vi "ReadINIandWriteToGFG.vi"(8 "error in (no error)":errorcluster, 10 "name or relative path":string="settings.ini", 11 "configuration file path":path) -> (0 "error out":errorcluster)   [LabVIEW 2012]
doc: "This VI reads an INI file and stores all keys in a Generalized Functional Global Variable (GFG). It then monitors updates to the GFG and writes keys back into INI file before closing. Note that the INI file only supports data type DBL or STRING. The GFG can handle any arbitrary data type, but values that are not DBL or STRING are discarded when closing and not written to INI file."
uses:
  String Array Operations/Check1DStringArrayForDuplicates.vi
  <vilib>/Utility/config.llb/Read Key (Double).vi
  <vilib>/Utility/config.llb/Read Key (String).vi
  <vilib>/Utility/config.llb/Read Key (Path).vi
  <vilib>/Utility/config.llb/NI_LVConfig.lvlib
  GFG/GFG library.lvlib
panel:
  out "error out 2":errorcluster
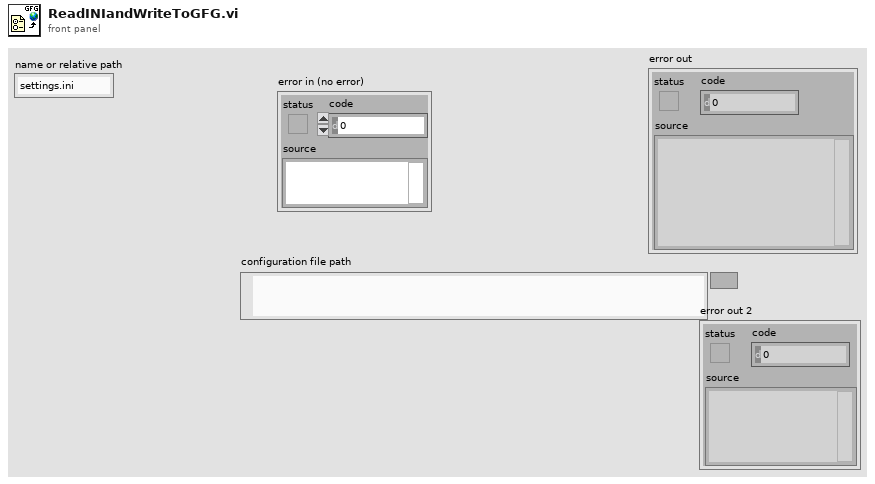
[diagram p1: front panel]
types:
  T1 = typedef "NI_LVConfig.lvlib/Config Data RefNum.ctl" = refnum<k1>
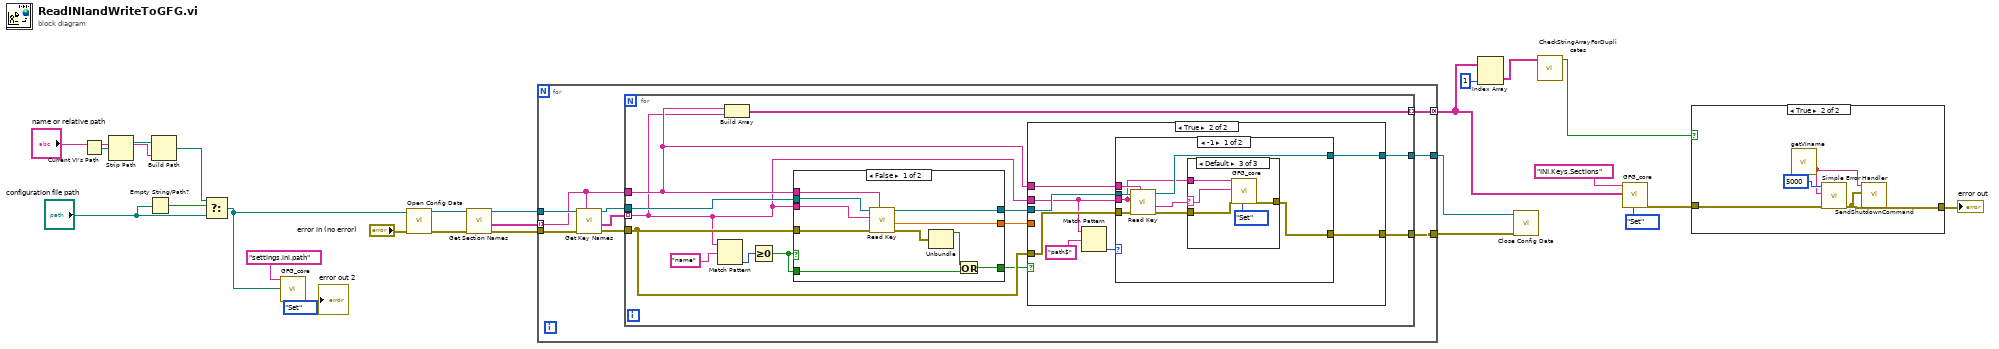
[diagram p0: block diagram]
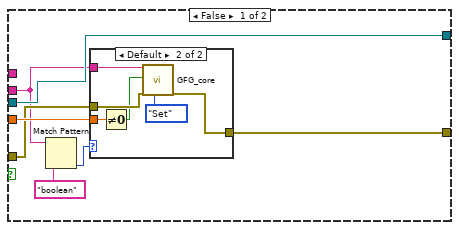
[diagram p4: hidden frame]
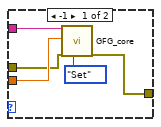
[diagram p5: hidden frame]
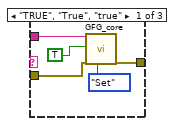
[diagram p6: hidden frame]
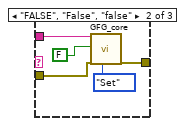
[diagram p7: hidden frame]
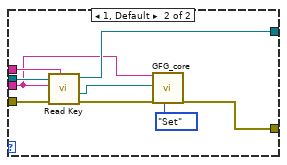
[diagram p8: hidden frame]
diagram:
  n1 = Current VI's Path() -> (path=w5:path)
  n2 = Strip Path(path=w5) -> (stripped path=w6:path)  [unwired: 1 out]
  n3 = Empty String/Path?(string/path="configuration file path") -> (empty?=w4:bool)
  n4 = Build Path(base path=w6, name or relative path="name or relative path") -> (appended path=w2:path)
  n5 = Select(t=w2, s=w4, f="configuration file path") -> (s? t:f=w1:path)
  n6 = call "GFG_core.vi"("Variable Name in"="settings.ini.path", "Variant in"=w1, "Action"=enum16{"Init", "Set", "Get"}."Set") -> ("error out"=→"error out 2":errorcluster)  [unwired: 10 in, 6 out]
  n7 = call <vilib>:"Open Config Data.vi"("error in (no error)"="error in (no error)", "configuration file path"=w1) -> ("error out"=w26:errorcluster, "refnum"=w25:T1)  [unwired: 7 in, 1 out]
  n8 = call <vilib>:"Get Section Names.vi"("error in (no error)"=w26, "refnum"=w25) -> ("error out"=w24:errorcluster, "section names"=w22:string[], "refnum out"=w23:T1)  [unwired: 7 in]
  n9 = for {
    tunnel: [w34] -> w21
    tunnel: w24 -> [w32]
    tunnel: w23 -> [w31]
    tunnel: w22 -> [w29] mode=indexing
    tunnel: [w28] -> w16 mode=concatenating
    tunnel: [w27] -> w20
    n10 = call <vilib>:"Get Key Names.vi"("section"=w29, "error in (no error)"=w32, "refnum"=w31) -> ("error out"=w33:errorcluster, "key names"=w35:string[], "refnum out"=w30:T1)  [unwired: 5 in, 1 out]
    n11 = for {
      tunnel: w30 -> [w48]
      tunnel: w29 -> [w42]
      tunnel: w35 -> [w39] mode=indexing
      tunnel: [w45] -> w34
      tunnel: w33 -> [w44]
      tunnel: [w43] -> w27
      tunnel: [w41] -> w28 mode=indexing
      n12 = Match Pattern(string=w39, regular expression="name") -> (offset past match=w38:i32)  [unwired: 1 in, 3 out]
      n13 = Build Array(w42, w39) -> (w41:string[])
      n14 = Greater Or Equal To 0?(x=w38) -> (x >= 0?=w36:bool)
      n15 = case shown="False" w36 {
        tunnel: w48 -> [w58 w60]
        tunnel: [w57 _] -> w47
        tunnel: [w56 w60] -> w46
        tunnel: w44 -> [w55 _]
        tunnel: w42 -> [w54 _]
        tunnel: w39 -> [w52 _]
        tunnel: w36 -> [w51 w59]
        tunnel: [w49 w59] -> w37
        frame False {
          n16 = call-poly <vilib>:"Read Key.vi"("section"=w54, "error in (no error)"=w55, "key"=w52, "refnum"=w58) -> ("error out"=w53:errorcluster, "value"=w57:dbl, "refnum out"=w56:T1)  [unwired: 4 in, 1 out]
          n17 = Unbundle(w53) -> ("status"=w50:bool)  [unwired: 2 out]
          n18 = Or(x=w50, y=w51) -> (x .or. y?=w49:bool)
        }
        frame True {
        }
      }
      n19 = case shown="True" w37 {
        tunnel: w47 -> [w66 _]
        tunnel: w39 -> [w61 w79]
        tunnel: w46 -> [w65 w86]
        tunnel: w42 -> [_ w85]
        tunnel: [w65 w84] -> w45
        tunnel: w44 -> [w64 w83]
        tunnel: [w67 w82] -> w43
        frame False {
          n20 = Match Pattern(string=w61, regular expression="boolean") -> (offset past match=w63:i32)  [unwired: 1 in, 3 out]
          n21 = case shown="Default" w63 {
            tunnel: w61 -> [w72 w78]
            tunnel: [w71 w77] -> w67
            tunnel: w66 -> [w69 w75]
            tunnel: w64 -> [w68 w74]
            frame -1 {
              n22 = call "GFG_core.vi"("Variable Name in"=w72, "Variant in"=w69, "error in (no error)"=w68, "Action"=enum16{"Init", "Set", "Get"}."Set") -> ("error out"=w71:errorcluster)  [unwired: 9 in, 6 out]
            }
            frame Default {
              n23 = Not Equal To 0?(x=w75) -> (x != 0?=w73:bool)
              n24 = call "GFG_core.vi"("Variable Name in"=w78, "Variant in"=w73, "error in (no error)"=w74, "Action"=enum16{"Init", "Set", "Get"}."Set") -> ("error out"=w77:errorcluster)  [unwired: 9 in, 6 out]
            }
          }
        }
        frame True {
          n25 = Match Pattern(string=w79, regular expression="path$") -> (offset past match=w81:i32)  [unwired: 1 in, 3 out]
          n26 = case shown="-1" w81 {
            tunnel: w86 -> [w94 w118]
            tunnel: w85 -> [w93 w117]
            tunnel: [w92 w116] -> w84
            tunnel: w83 -> [w91 w115]
            tunnel: [w89 w110] -> w82
            tunnel: w79 -> [w87 w112]
            frame -1 {
              n27 = call-poly <vilib>:"Read Key.vi"("section"=w93, "error in (no error)"=w91, "key"=w87, "refnum"=w94) -> ("error out"=w90:errorcluster, "value"=w88:string, "refnum out"=w92:T1)  [unwired: 4 in, 1 out]
              n28 = case shown="Default" w88 {
                selector: w88 -> [_ _ w105]
                tunnel: w87 -> [w99 w104 w109]
                tunnel: w90 -> [w97 w102 w107]
                tunnel: [w96 w101 w106] -> w89
                frame "TRUE", "True", "true" {
                  n29 = call "GFG_core.vi"("Variable Name in"=w99, "Variant in"=TRUE, "error in (no error)"=w97, "Action"=enum16{"Init", "Set", "Get"}."Set") -> ("error out"=w96:errorcluster)  [unwired: 9 in, 6 out]
                }
                frame "FALSE", "False", "false" {
                  n30 = call "GFG_core.vi"("Variable Name in"=w104, "Variant in"=FALSE, "error in (no error)"=w102, "Action"=enum16{"Init", "Set", "Get"}."Set") -> ("error out"=w101:errorcluster)  [unwired: 9 in, 6 out]
                }
                frame Default {
                  n31 = call "GFG_core.vi"("Variable Name in"=w109, "Variant in"=w105, "error in (no error)"=w107, "Action"=enum16{"Init", "Set", "Get"}."Set") -> ("error out"=w106:errorcluster)  [unwired: 9 in, 6 out]
                }
              }
            }
            frame 1, Default {
              n32 = call-poly <vilib>:"Read Key.vi"("section"=w117, "error in (no error)"=w115, "key"=w112, "refnum"=w118) -> ("error out"=w114:errorcluster, "value"=w113:path, "refnum out"=w116:T1)  [unwired: 4 in, 1 out]
              n33 = call "GFG_core.vi"("Variable Name in"=w112, "Variant in"=w113, "error in (no error)"=w114, "Action"=enum16{"Init", "Set", "Get"}."Set") -> ("error out"=w110:errorcluster)  [unwired: 9 in, 6 out]
            }
          }
        }
      }
    }
  }
  n34 = Index Array(array=w16, index (col)=1 ("disabled index (col)")) -> (element=w14:string[])  [unwired: 1 in]
  n35 = call <vilib>:"Close Config Data.vi"("error in (no error)"=w20, "refnum"=w21) -> ()  [unwired: 8 in, 2 out]
  n36 = call-poly "CheckStringArrayForDuplicates.vi"("String Array"=w14) -> ("duplicate string found?"=w13:bool)  [unwired: 10 in]
  n37 = call "GFG_core.vi"("Variable Name in"="INI.Keys.Sections", "Variant in"=w16, "Action"=enum16{"Init", "Set", "Get"}."Set") -> ("error out"=w12:errorcluster)  [unwired: 10 in, 6 out]
  n38 = case shown="True" w13 {
    tunnel: w12 -> [w119 w122]
    tunnel: [w119 w120] -> w11
    frame False {
    }
    frame True {
      n39 = call "getVIname.vi"() -> ("VI name"=w121:string)  [unwired: 19 in]
      n40 = call <vilib>:"Simple Error Handler.vi"("error code (no error:0)"=5000, "error source (\" \")"=w121, "error in (no error)"=w122) -> ("error out"=w120:errorcluster)  [unwired: 2 in, 4 out]
      n41 = call "SendShutdownCommand.vi"("dummy input"=w120, "Source VI"=w121) -> ()  [unwired: 10 in]
    }
  }
  "error out" <- w11
